vi "ASDA-A2_PR Event_Path Setting.vi"(8 "error in":errorcluster, 10 "Path Setting":T1={"Command"=enum."Absolute", "Position"=0, "Speed"=1}, 11 "Buffer Data In":T2) -> (0 "error out":errorcluster, 3 "Buffer Data Out":T2)   [LabVIEW 2016]
uses:
  Data Def/ASDA-A2_Buffer Data.ctl
  Data Def/ASDA-A2_Write Register Data.ctl
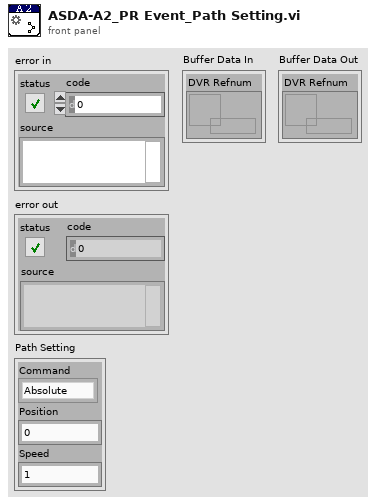
[diagram p1: front panel]
types:
  T1 = cluster{"Command":enum16{"Absolute", "Increase", "Relative"}, "Position":i32, "Speed":u16}
  T2 = typedef "ASDA-A2_Buffer Data.ctl" = cluster{"DVR Refnum":refnum<data-value>}
  T3 = typedef "ASDA-A2_Write Register Data.ctl" = cluster{"Address":u16, "Max Value":u32, "Min Value":u32, "Value":u32, "Type":enum16{"16 Bits", "32 Bits"}, "Page":string, "Description":string}
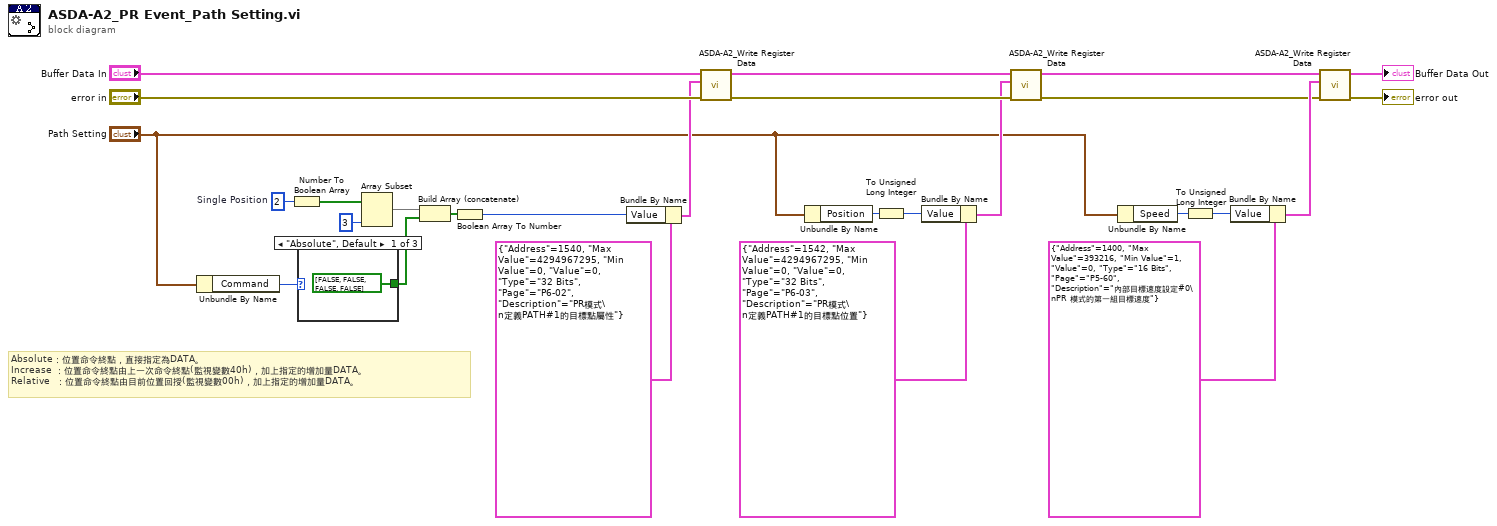
[diagram p0: block diagram]
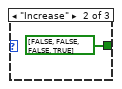
[diagram p2: hidden frame]
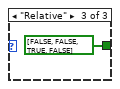
[diagram p3: hidden frame]
diagram:
  w27 = u8 2  # Single Position
  # "Absolute：位置命令終點，直接指定為DATA。\nIncrease ：位置命令終點由上一次命令終點(監視變數40h)，加上指定的增加量DATA。\nRelative  ：位置命令終點由目前位置回授(監視變數00h)，加上指定的增加量DATA。"
  n1 = Unbundle By Name("Path Setting") -> ("Command"=w24:enum16{"Absolute", "Increase", "Relative"})
  n2 = Number To Boolean Array(number=w27) -> (Boolean array=w26:bool[])
  n3 = case shown="\"Absolute\", Default" w24 {
    tunnel: [bool[] [FALSE, FALSE, FALSE, FALSE] bool[] [FALSE, FALSE, FALSE, TRUE] bool[] [FALSE, FALSE, TRUE, FALSE]] -> w22
    frame "Absolute", Default {
    }
    frame "Increase" {
    }
    frame "Relative" {
    }
  }
  n4 = Array Subset(array=w26, length=3) -> (w23:bool[])  [unwired: 1 in]
  n5 = Build Array (concatenate)(w23, w22) -> (w21:bool[])
  n6 = Boolean Array To Number(Boolean array=w21) -> (number=w19:u32)
  n7 = Bundle By Name(cluster=T3 {"Address"=1540, "Max Value"=4294967295, "Min Value"=0, "Value"=0, "Type"=enum."32 Bits", "Page"="P6-02", "Description"="PR模式\n定義PATH#1的目標點屬性"} ("Write Register Data"), "Value"=w19) -> (w17:T3)
  n8 = call "ASDA-A2_Write Register Data.vi"("error in"="error in", "Write Register Data"=w17, "Buffer Data In"="Buffer Data In") -> ("error out"=w15:errorcluster, "Buffer Data Out"=w14:T2)  [unwired: 7 in]
  n9 = Unbundle By Name("Path Setting") -> ("Position"=w13:i32)
  n10 = To Unsigned Long Integer(number=w13) -> (unsigned 32bit integer=w12:u32)
  n11 = Bundle By Name(cluster=T3 {"Address"=1542, "Max Value"=4294967295, "Min Value"=0, "Value"=0, "Type"=enum."32 Bits", "Page"="P6-03", "Description"="PR模式\n定義PATH#1的目標點位置"} ("Write Register Data"), "Value"=w12) -> (w10:T3)
  n12 = call "ASDA-A2_Write Register Data.vi"("error in"=w15, "Write Register Data"=w10, "Buffer Data In"=w14) -> ("error out"=w5:errorcluster, "Buffer Data Out"=w4:T2)  [unwired: 7 in]
  n13 = Unbundle By Name("Path Setting") -> ("Speed"=w6:u16)
  n14 = To Unsigned Long Integer(number=w6) -> (unsigned 32bit integer=w7:u32)
  n15 = Bundle By Name(cluster=T3 {"Address"=1400, "Max Value"=393216, "Min Value"=1, "Value"=0, "Type"=enum."16 Bits", "Page"="P5-60", "Description"="內部目標速度設定#0\nPR 模式的第一組目標速度"} ("Write Register Data"), "Value"=w7) -> (w9:T3)
  n16 = call "ASDA-A2_Write Register Data.vi"("error in"=w5, "Write Register Data"=w9, "Buffer Data In"=w4) -> ("error out"=→"error out":errorcluster, "Buffer Data Out"=→"Buffer Data Out":T2)  [unwired: 7 in]
